vi "DFD FXP NStage MRate Postprocessing (I16, nCh).vi"(5 "input range":dbl=1.0, 6 "history in":i16[](array[numeric]), 7 "# channels":i32=1, 8 "error in (no error)":errorcluster, 10 "multirate filters":T1[](array[typedef]) {"mMRate_SumWl" min=1 max=32 step=1; "mMRate_InputIwl" min=1 max=32 step=1; "mMRate_GainWl" min=1 max=32 step=1; "mMRate_OutputWl" min=1 max=32 step=1; "mMRate_InputWl" min=1 max=32 step=1; "mMRate_CoefWl" min=1 max=32 step=1; "mMRate_Mode" items=["Default"=-1, "No Rate Change"=0, "Interpolation"=1, "Decimation"=2, "Interpolated"=3, "Rational"=4]}, 11 "signal in":i16[](array[numeric]) format="%.0x") -> (0 "error out":errorcluster, 3 "signal out":dbl[][](array[numeric]), 4 "history out":i16[](array[numeric]))   [LabVIEW 2017, in "NI_DigFilterLicensed.lvlib"]
doc: "Converts the output signal of a fixed-point multistage multirate filter from a fixed-point representation to a floating-point representation. You must manually select the polymorphic instance you want to use."
uses:
  <vilib>/addons/Digital Filter Design/NI_DigFilterLicensed.lvlib
  <vilib>/addons/Digital Filter Design/_Objects.llb/DFD Multirate Filter Obj.ctl
  <vilib>/addons/Digital Filter Design/_Objects.llb/DFD Multirate Mode.ctl
  <vilib>/addons/Digital Filter Design/_Objects.llb/DFD Coef Norm Type.ctl
  <vilib>/addons/Digital Filter Design/_Objects.llb/DFD Round-off Mode.ctl
  <vilib>/addons/Digital Filter Design/_Objects.llb/DFD FXP MRate Multiply Mode.ctl
  <vilib>/addons/Digital Filter Design/_Misc.llb/dfd_Error Handlers (Single).vi
  <vilib>/addons/Digital Filter Design/NI_DigFilter_FXP.lvlib
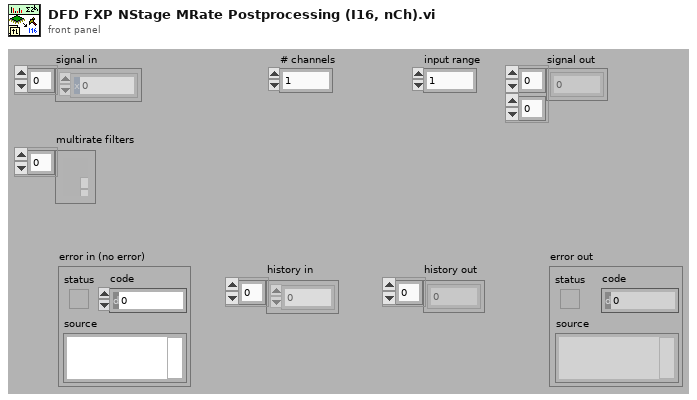
[diagram p1: front panel]
types:
  T1 = typedef "NI_DigFilterLicensed.lvlib/DFD Multirate Filter Obj.ctl" = cluster{"mMRate_Structure":enum16{"CIC", "FIR", "IIR", "Lattice"}, "mMRate_Mode":T2, "mMRate_Factor":i32, "mMRate_FIRParams":cluster{"mMRate_FIR_H":dbl[], "mMRate_FIR_IsNyquist?":bool, "mMRate_FIR_IsSymmetric?":bool}, "mMRate_CICParams":cluster{"mMRate_CIC_#Stage":i32, "mMRate_CIC_Lag":i32, "mMRate_CIC_Type":enum16{"Lowpass", "Highpass"}}, "mMRate_Order":i32, "mMRate_Version":string, "mMRate_Comments":string, "mMRate_RationalFactor":cluster{"mMRate_L":i32, "mMRate_M":i32}, "mMRate_Fs":dbl, "mMRate_Quantized?":bool, "mMRate_QFilterGain":dbl, "mMRate_CoefWl":i16, "mMRate_Scaling":cluster{"mMRate_ScaleByPowerOf2?":bool, "mMRate_ScaleType":T3}, "mMRate_InputWl":i16, "mMRate_OutputWl":i16, "mMRate_OutputMode":T4, "mMRate_MultMode":T5, "mMRate_BitPruning":bool, "mMRate_GainWl":i16, "mMRate_OutputFwl":i16, "mMRate_SumIwl":i16, "mMRate_InputIwl ":i16, "mMRate_SumWl":i16, "mMRate_CoefIwl":i16}
  T2 = typedef "NI_DigFilterLicensed.lvlib/DFD Multirate Mode.ctl" = i16
  T3 = typedef "NI_DigFilterLicensed.lvlib/DFD Coef Norm Type.ctl" = enum16{"No Norm", "Time Domain 1-Norm", "Time Domain 2-Norm", "Time Domain Inf-Norm"}
  T4 = typedef "NI_DigFilterLicensed.lvlib/DFD Round-off Mode.ctl" = enum16{"Nearest", "Truncation"}
  T5 = typedef "NI_DigFilterLicensed.lvlib/DFD FXP MRate Multiply Mode.ctl" = enum16{"Truncated", "Full"}
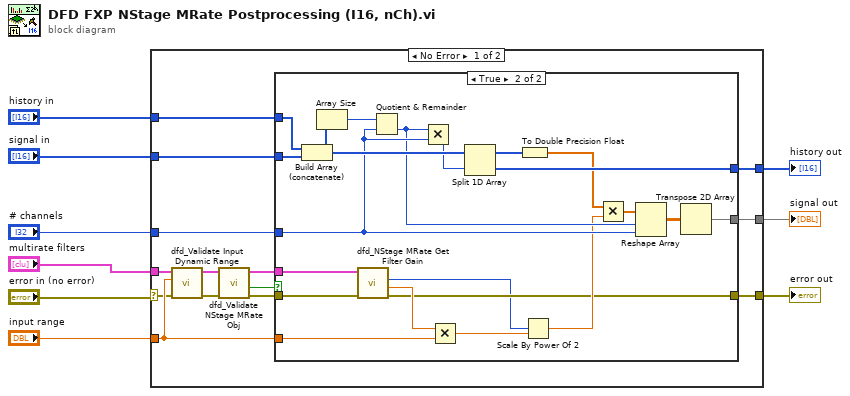
[diagram p0: block diagram]
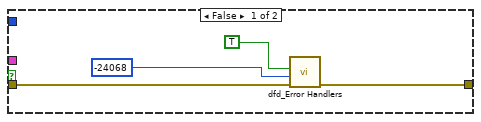
[diagram p2: hidden frame]
diagram:
  n1 = case shown="No Error" "error in (no error)" {
    selector: "error in (no error)" -> [w10 w47]
    tunnel: [w21 w47] -> w9
    tunnel: "# channels" -> [w20 _]
    tunnel: "signal in" -> [w19 _]
    tunnel: "history in" -> [w18 _]
    tunnel: [w17 _] -> w5
    tunnel: [w16 _] -> w4
    tunnel: "input range" -> [w13 _]
    tunnel: "multirate filters" -> [w12 _]
    frame No Error {
      n2 = call <vilib>:"dfd_Validate Input Dynamic Range.vi"("error in (no error)"=w10, "input range"=w13) -> ("error out"=w14:errorcluster)  [unwired: 9 out]
      n3 = call <vilib>:"dfd_Validate NStage MRate Obj.vi"("error in"=w14, "multirate filters"=w12) -> ("error out"=w11:errorcluster, "is valid FXP?"=w15:bool, "dup multirate filters"=w22:T1[])  [unwired: 7 out]
      n4 = case shown="True" w15 {
        tunnel: w19 -> [_ w45]
        tunnel: w18 -> [_ w44]
        tunnel: [_ w41] -> w17
        tunnel: [_ w38] -> w16
        tunnel: w20 -> [_ w37]
        tunnel: w22 -> [_ w30]
        tunnel: w13 -> [_ w29]
        tunnel: w11 -> [w24 w28]
        tunnel: [w23 w28] -> w21
        frame False {
          n5 = call-poly <vilib>:"dfd_Error Handlers.vi"("error in (no error)"=w24, "error code"=-24068 ("ERR_INVALID_FXP_MRATE"), "condition failed?"=TRUE) -> ("error out"=w23:errorcluster)  [unwired: 8 out]
        }
        frame True {
          n6 = Build Array (concatenate)(w44, w45) -> (w43:i16[])
          n7 = Array Size(array=w43) -> (size(s)=w46:i32)
          n8 = call <vilib>:"dfd_NStage MRate Get Filter Gain.vi"("multirate filters"=w30) -> ("gain"=w31:dbl, "NStage output -fwl"=w27:i16)  [unwired: 9 out]
          n9 = Quotient & Remainder(x=w46, y=w37) -> (floor(x/y)=w36:i32)  [unwired: 1 out]
          n10 = Multiply(x=w36, y=w37) -> (x*y=w42:i32)
          n11 = Multiply(x=w31, y=w29) -> (x*y=w34:dbl)
          n12 = Split 1D Array(array=w43, index=w42) -> (first subarray=w35:i16[], second subarray=w41:i16[])
          n13 = To Double Precision Float(number=w35) -> (double precision float=w33:dbl[])
          n14 = Scale By Power Of 2(n=w27, x=w34) -> (x*2^n=w32:dbl)
          n15 = Multiply(x=w33, y=w32) -> (x*y=w40:dbl[])
          n16 = Reshape Array(w40, w36, w37) -> (w39:dbl[][])
          n17 = Transpose 2D Array(2D array=w39) -> (transposed array=w38:dbl[][])
        }
      }
    }
    frame Error {
    }
  }
  "signal out" <- w4
  "error out" <- w9
  "history out" <- w5
